vi "write command and read multiple.vi"(8 "error in (no error)":errorcluster, 10 "Read Actual\nPosition":string, 11 "VISA Refnum in":refnum<visa-resource-name>) -> (0 "error out":errorcluster, 2 "Array":string[](array[string]), 3 "VISA Refnum out":refnum<visa-resource-name>)   [LabVIEW 2013]
panel:
  out "Array 2":errorcluster[](array[cluster])
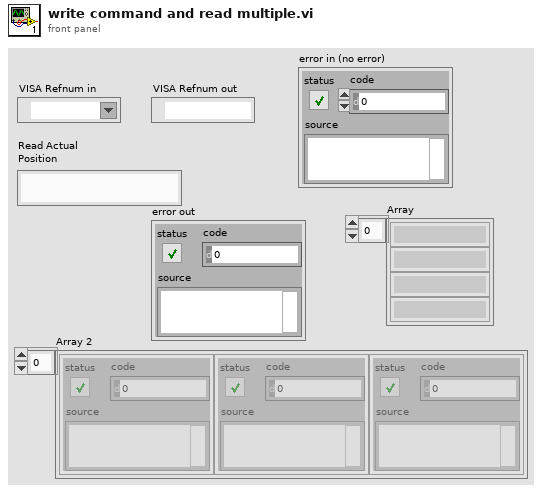
[diagram p1: front panel]
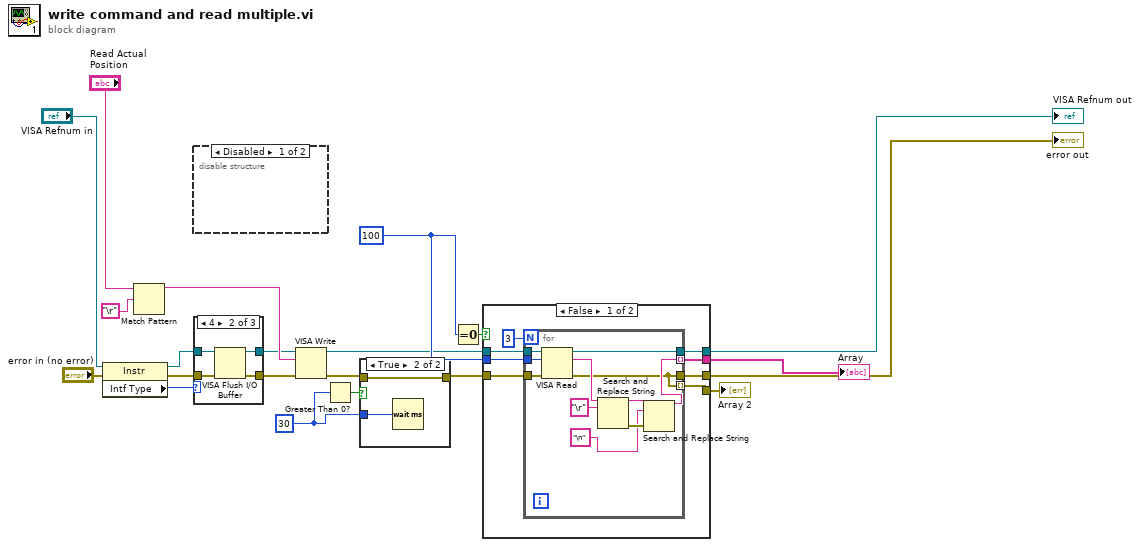
[diagram p0: block diagram]
diagram:
  w8 = u32 30 ("Wait before read (0ms)")
  w10 = u32 100 ("Bytes to read (100)")
  n1 = property class="Instr"(reference="VISA Refnum in", error in="error in (no error)") -> (reference out=w13:refnum<visa-resource-name>, error out=w14:errorcluster, "Intf Type"=w12:u16)
  n2 = Match Pattern(string="Read Actual\nPosition", regular expression="\r") -> (before substring=w16:string)  [unwired: 4 out]
  n3 = disable-structure shown="Disabled" {
    frame Disabled {
    }
    frame Enabled {
    }
  }
  n4 = case shown="4" w12 {
    tunnel: w13 -> [w23 w25 w29]
    tunnel: [w23 w24 w29] -> w4
    tunnel: w14 -> [w22 w27 w28]
    tunnel: [w22 w26 w28] -> w5
    frame 1 {
    }
    frame 4 {
      n5 = VISA Flush I/O Buffer(VISA resource name=w25, error in (no error)=w27) -> (VISA resource name out=w24:refnum<visa-resource-name>, error out=w26:errorcluster)  [unwired: 1 out]
    }
    frame Default {
    }
  }
  n6 = VISA Write(VISA resource name=w4, write buffer=w16, error in (no error)=w5) -> (VISA resource name out=w3:refnum<visa-resource-name>, error out=w6:errorcluster)  [unwired: 1 out]
  n7 = Greater Than 0?(x=w8) -> (x > 0?=w9:bool)
  n8 = case shown="True" w9 {
    tunnel: w6 -> [w30 w32]
    tunnel: [w30 w32] -> w7
    tunnel: w8 -> [_ w31]
    frame False {
    }
    frame True {
      n9 = Wait (ms)(milliseconds to wait=w31) -> ()  [unwired: 1 out]
    }
  }
  n10 = Equal To 0?(x=w10) -> (x = 0?=w11:bool)
  n11 = case shown="False" w11 {
    tunnel: [w40 w53] -> w20
    tunnel: w3 -> [w39 w52]
    tunnel: [w38 w52] -> w19
    tunnel: w10 -> [w37 _]
    tunnel: [w36 _] -> w21
    tunnel: w7 -> [w35 w53]
    tunnel: [w33 _] -> w1
    frame False {
      n12 = for {
        N: 3 -> [_]
        tunnel: [w41] -> w40
        tunnel: w39 -> [w51]
        tunnel: [w50] -> w38
        tunnel: w37 -> [w49]
        tunnel: [w43] -> w36 mode=indexing
        tunnel: w35 -> [w48]
        tunnel: [w41] -> w33 mode=indexing
        n13 = VISA Read(VISA resource name=w51, byte count=w49, error in (no error)=w48) -> (VISA resource name out=w50:refnum<visa-resource-name>, read buffer=w46:string, error out=w41:errorcluster)  [unwired: 1 out]
        n14 = Search and Replace String(input string=w46, search string="\r") -> (result string=w45:string, error out=w44:errorcluster)  [unwired: 6 in, 2 out]
        n15 = Search and Replace String(input string=w45, search string="\n", error in=w44) -> (result string=w43:string)  [unwired: 5 in, 3 out]
      }
    }
    frame True {
    }
  }
  "Array" <- w21
  "error out" <- w20
  "VISA Refnum out" <- w19
  "Array 2" <- w1
